vi "Create Enable Periodic.vi"(8 "error in (no error)":errorcluster, 10 "Channel Parameters":T2, 11 "Message Channels Section in":T1 format="%.0x") -> (0 "error out":errorcluster, 3 "Message Channels Section out":T1 format="%.0x")   [LabVIEW 2020, in "Instrument Addon Scripting API.lvlib"]
uses:
  Instrument Addon Scripting API.lvlib
  <vilib>/NI VeriStand/Custom Device API/Custom Device Item Ref.ctl
  <vilib>/NI VeriStand/Custom Device API/Custom Device Channel.ctl
  <vilib>/NI VeriStand/Custom Device API/Custom Device Channel Type.ctl
  Addon/Addon Shared/SubVIs/Constants.vi
  Addon/Addon Shared/Instrument Addon Shared.lvlib
  <vilib>/NI VeriStand/Custom Device API/Custom Device API.lvlib
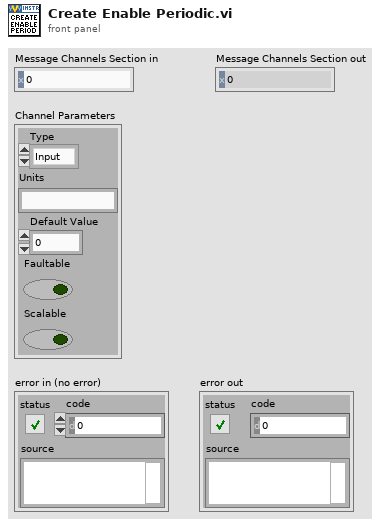
[diagram p1: front panel]
types:
  T1 = typedef "Custom Device API.lvlib/Custom Device Item Ref.ctl" = u64
  T2 = typedef "Custom Device API.lvlib/Custom Device Channel.ctl" = cluster{"Type":T3, "Units":string, "Default Value":dbl, "Faultable":bool, "Scalable":bool}
  T3 = typedef "Custom Device API.lvlib/Custom Device Channel Type.ctl" = enum16{"Input", "Output"}
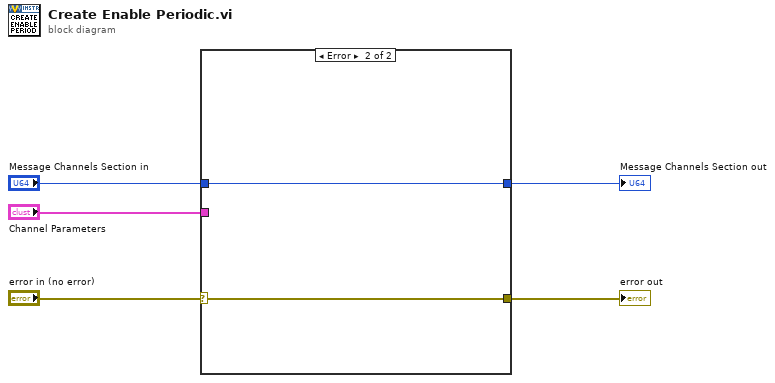
[diagram p0: block diagram]
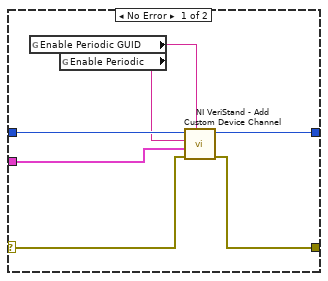
[diagram p2: hidden frame]
diagram:
  n1 = case shown="Error" "error in (no error)" {
    selector: "error in (no error)" -> [w6 w13]
    tunnel: "Message Channels Section in" -> [w12 w14]
    tunnel: [w11 w13] -> w4
    tunnel: "Channel Parameters" -> [w10 _]
    tunnel: [w7 w14] -> w2
    frame No Error {
      n2 = global read "Constants.vi" "Enable Periodic GUID"() -> (w8:string)
      n3 = global read "Constants.vi" "Enable Periodic"() -> (w9:string)
      n4 = call <vilib>:"NI VeriStand - Add Custom Device Channel.vi"("GUID (Default Channel)"=w8, "error in (no error)"=w6, "Channel"=w10, "Channel Name"=w9, "Parent Ref in"=w12) -> ("error out"=w11:errorcluster, "Parent Ref out"=w7:T1)  [unwired: 3 in, 2 out]
    }
    frame Error {
    }
  }
  "error out" <- w4
  "Message Channels Section out" <- w2
